vi "get_settings_cluster.vi"(8 "error in (no error)":errorcluster, 11 "GenericPlugin in":refnum<class "GenericClock.lvclass">) -> (0 "error out":errorcluster, 2 "settings cluster":variant, 3 "GenericPlugin out":refnum<class "GenericClock.lvclass">)   [LabVIEW 2010, in "GenericClock.lvclass"]
uses:
  GenericClock.lvclass
  GenericClock.lvclass/GenericClock.ctl
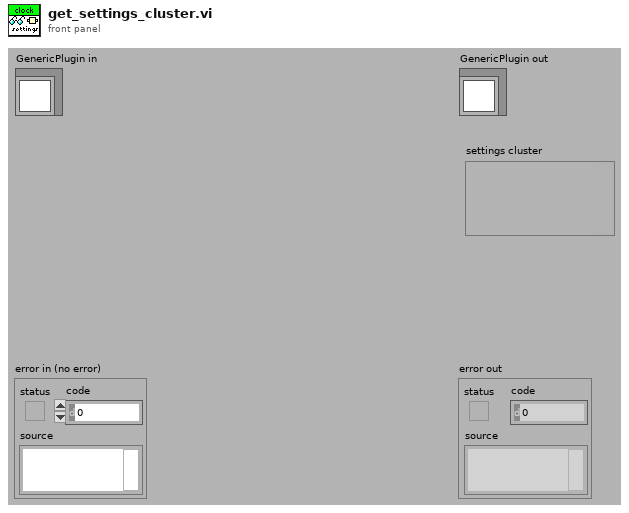
[diagram p1: front panel]
types:
  T1 = typedef "GenericClock.lvclass/settings_cluster.ctl" = cluster{"frequency":dbl[unit], "number of cycles":i32, "offset":dbl[unit], "base frequency":dbl[unit], "gate high duration":dbl[unit], "duty cycle":dbl[unit], "triggered?":bool}
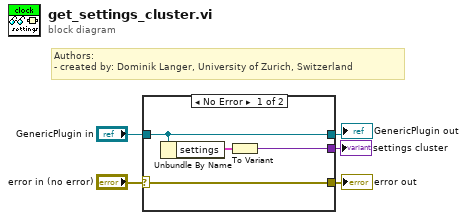
[diagram p0: block diagram]
diagram:
  # "Authors: \n- created by: Dominik Langer, University of Zurich, Switzerland"
  n1 = case shown="No Error" "error in (no error)" {
    selector: "error in (no error)" -> [w6 w11]
    tunnel: "GenericPlugin in" -> [w9 w10]
    tunnel: [w7 _] -> w3
    tunnel: [w6 w11] -> w2
    tunnel: [w9 w10] -> w1
    frame No Error {
      n2 = Unbundle By Name(w9) -> ("settings"=w8:T1)
      n3 = To Variant(anything=w8) -> (Variant=w7:variant)
    }
    frame Error {
    }
  }
  "error out" <- w2
  "GenericPlugin out" <- w1
  "settings cluster" <- w3
